vi "ManipStopIntaking.vi"() -> (0 "Error Out":errorcluster, 1 "Advance Trigger":bool)   [LabVIEW 2023]
doc: "This VI switches whether the robot intake is on or off in autonomous.\n\nParameters:\n1. \"on\" or \"off\""
uses:
  GlobalNoteHandling.vi
  GlobalDriverStationCommands.vi
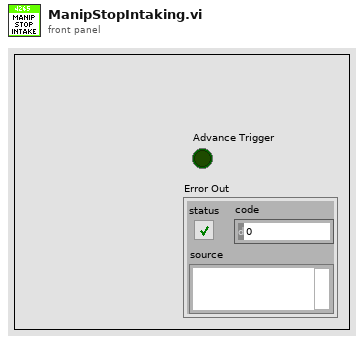
[diagram p1: front panel]
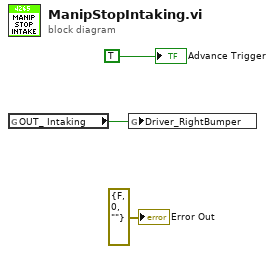
[diagram p0: block diagram]
diagram:
  n1 = global read "GlobalNoteHandling.vi" "OUT_ Intaking"() -> (w2:bool)
  n2 = global write "GlobalDriverStationCommands.vi" "Driver_RightBumper"(w2) -> ()
  "Advance Trigger" <- TRUE
  "Error Out" <- errorcluster {"status"=FALSE, "code"=0, "source"=""} ("Error Out")
